vi "Test - 4.vi"() -> ()   [LabVIEW 2013]
uses:
  Channel/Ctls/ChannelSetting.ctl
  Channel/Ctls/IOType.ctl
  Channel/Ctls/Dimensions.ctl
  Section/Section.lvclass
  Channel/Channel.lvclass
  Generic/Generic.lvclass
  Item/Item.lvclass
  Item/Ctls/Item Reference.ctl
  <vilib>/NI Veristand/Custom Device API/Custom Device API.lvlib
panel:
  out "Property Names 2":string[](array[string])
  out "x = y?":bool
  out "PathName 2":string
  out "TagGUID":string
  out "Description":string
  out "PathName":string
  out "Property Names":string[](array[string])
  out "x-y":u32
  out "Request invalid?":bool
  out "Channels":T4(array[cluster])
  out "数组":T5(array[cluster])
  out "Value 2":variant
  # "19999"
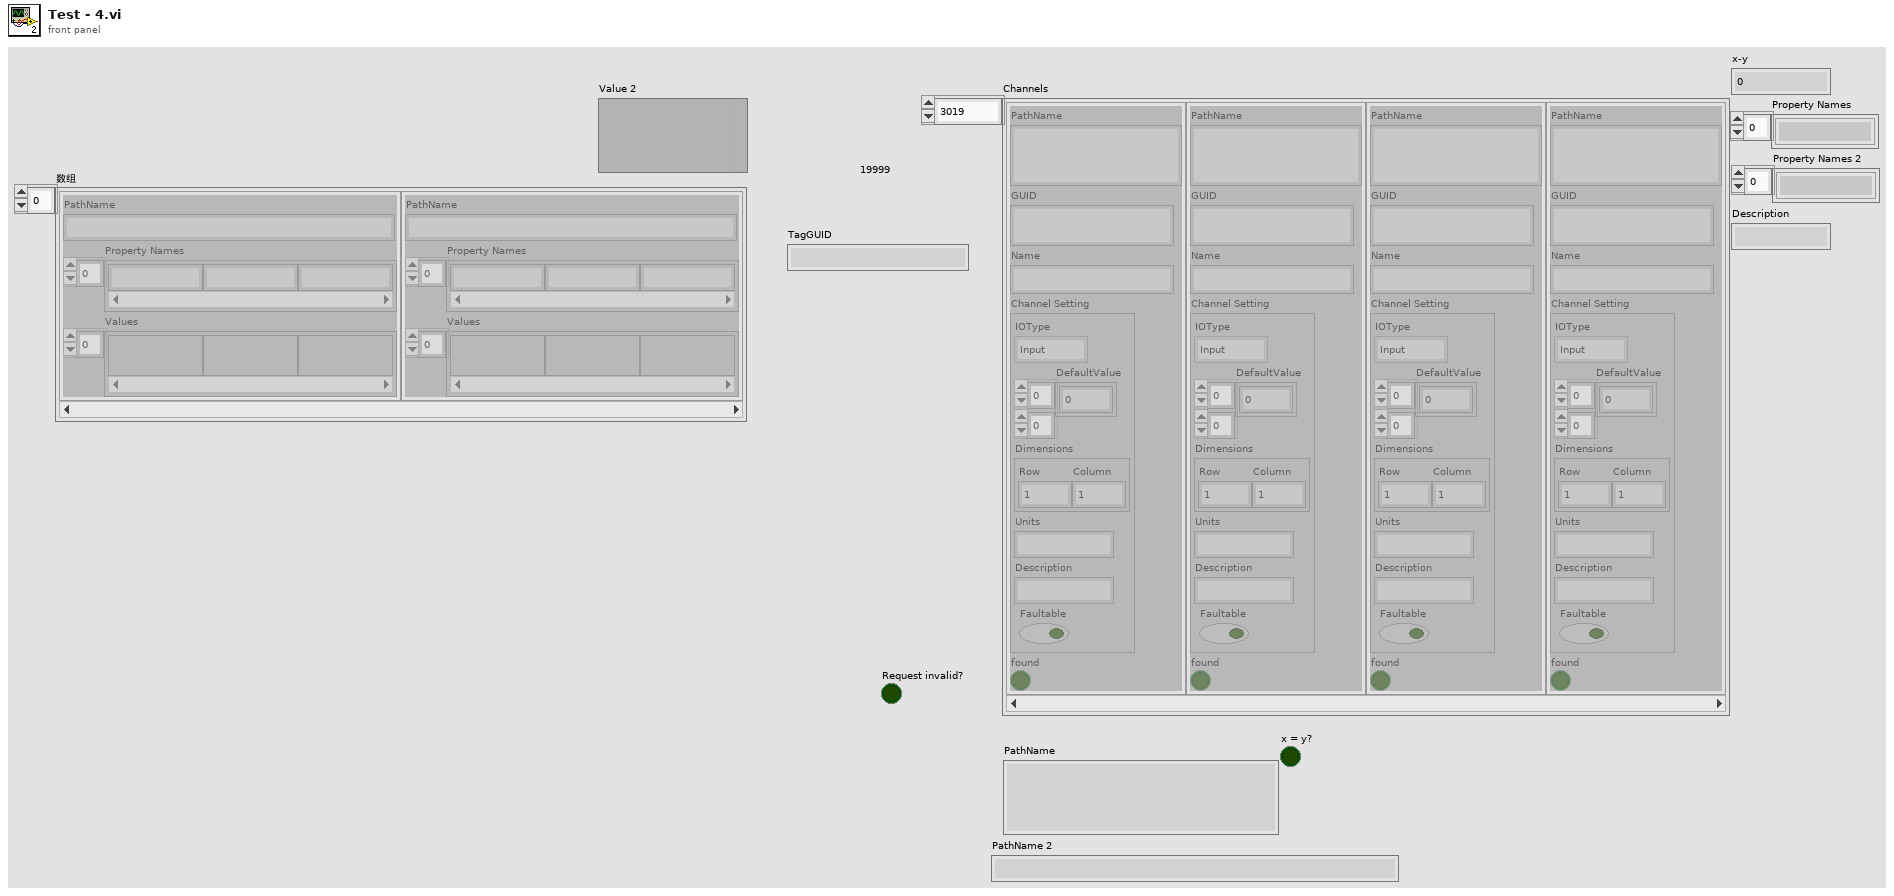
[diagram p1: front panel]
types:
  T1 = typedef "Hierarchy Framework.lvlib/Channel.lvclass/ChannelSetting.ctl" = cluster{"IOType":T2, "DefaultValue":dbl[][], "Dimensions":T3, "Units":string, "Description":string, "Faultable":bool}
  T2 = typedef "Hierarchy Framework.lvlib/Channel.lvclass/IOType.ctl" = enum16{"Input", "Output"}
  T3 = typedef "Hierarchy Framework.lvlib/Channel.lvclass/Dimensions.ctl" = cluster{"Row":i32, "Column":i32}
  T4 = cluster{"PathName":string, "GUID":string, "Name":string, "Channel Setting":T1, "found":bool}[]
  T5 = cluster{"PathName":string, "Property Names":string[], "Values":variant[]}[]
  T6 = typedef "Hierarchy Framework.lvlib/Item.lvclass/Item Reference.ctl" = u64
  T7 = cluster{"Accessors:PathName":string, "Property Names":string[], "Values":variant[]}
  T8 = cluster{"PathName":string, "GUID":string, "Name":string, "ChannelSetting":T1, "found":bool}
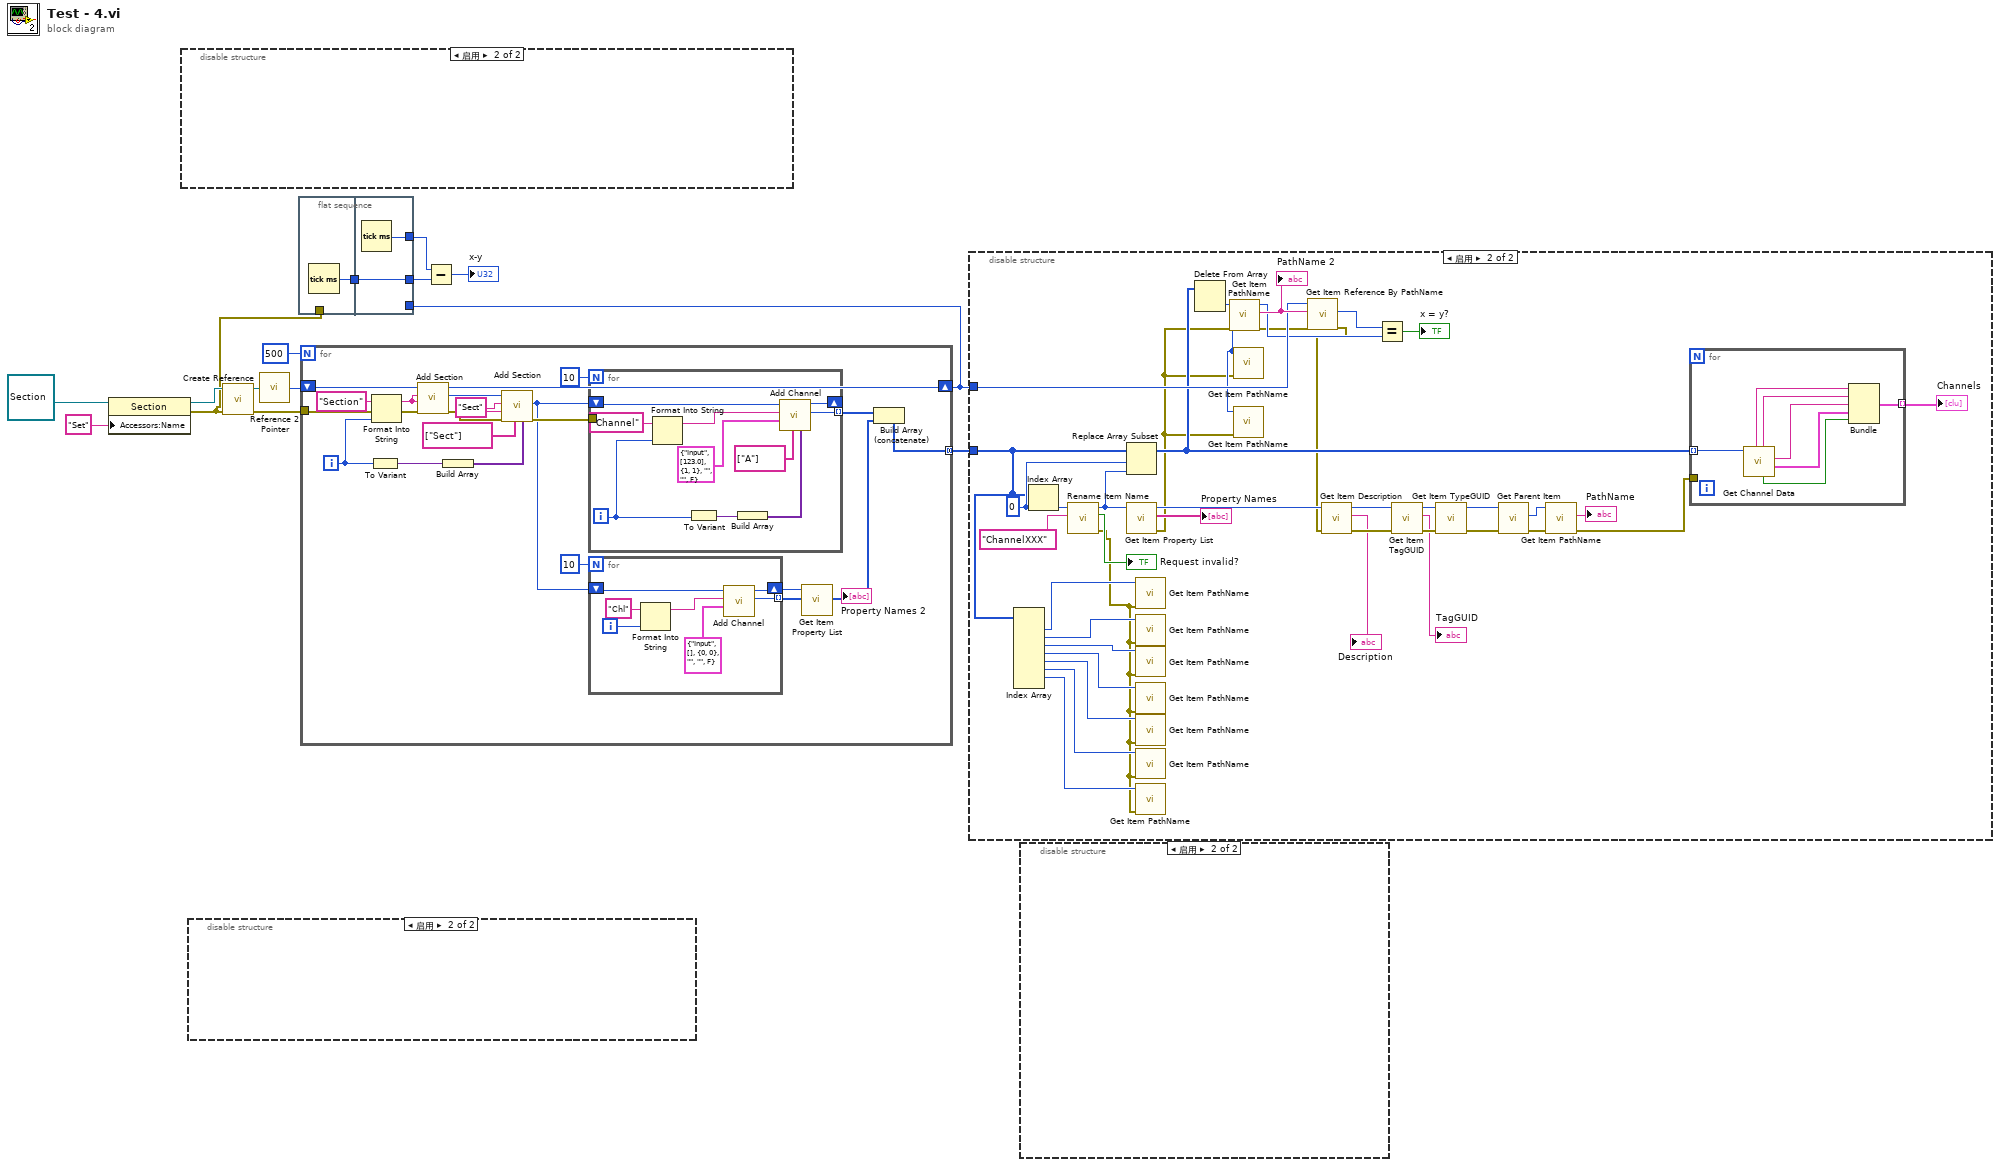
[diagram p0: block diagram]
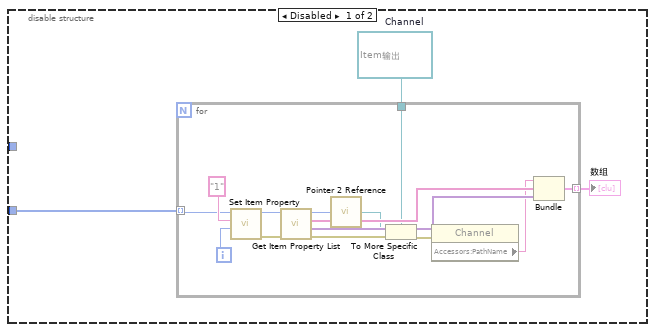
[diagram p2: hidden frame]
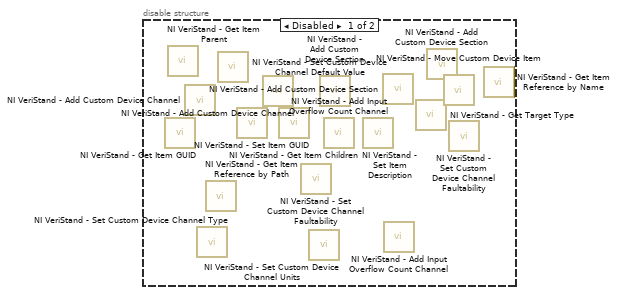
[diagram p3: hidden frame]
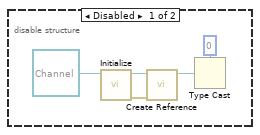
[diagram p4: hidden frame]
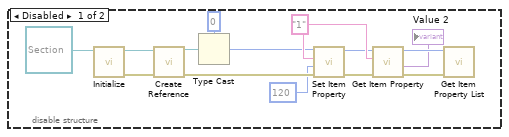
[diagram p5: hidden frame]
diagram:
  n1 = property class="Section"(reference=refnum<class "Section.lvclass"> refnum ("Framework.lvlib:Section"), "Accessors:Name"="Set" ("Name")) -> (reference out=w12:refnum<class "Section.lvclass">, error out=w8:errorcluster)  [unwired: 1 in]
  n2 = disable-structure shown="启用" {
    frame Disabled {
      n3 = call-dynamic "Initialize.vi"("Channel输入"=refnum<class "Channel.lvclass"> refnum ("Framework.lvlib:Channel")) -> ("error out"=w17:errorcluster, "Channel输出"=w18:refnum<class "Channel.lvclass">)  [unwired: 9 in]
      n4 = call "Create Reference.vi"("error in (no error)"=w17, "Generic"=w18) -> ("Generic Reference"=w16:refnum<data-value>)  [unwired: 8 in, 1 out]
      n5 = Type Cast(type=T6 0 ("Item Reference out"), x=w16) -> ()  [unwired: 1 out]
    }
    frame Enabled {
    }
  }
  n6 = disable-structure shown="启用" {
    frame Disabled {
      w31 = "1" ("Property Name")
      n7 = call-dynamic "Initialize.vi"("Section输入"=refnum<class "Section.lvclass"> refnum ("Framework.lvlib:Section")) -> ("error out"=w23:errorcluster, "Section输出"=w24:refnum<class "Section.lvclass">)  [unwired: 9 in]
      n8 = call "Create Reference.vi"("error in (no error)"=w23, "Generic"=w24) -> ("error out"=w29:errorcluster, "Generic Reference"=w21:refnum<data-value>)  [unwired: 8 in]
      n9 = Type Cast(type=T6 0 ("Item Reference out"), x=w21) -> (*(type *) &x=w20:T6)
      n10 = call "Set Item Property.vi"("error in (no error)"=w29, "Value"=u64 120 ("Generic Reference"), "Property Name"=w31, "Item Reference in"=w20) -> ("error out"=w28:errorcluster, "Item Reference out"=w30:T6)  [unwired: 5 in, 1 out]
      n11 = call "Get Item Property.vi"("error in (no error)"=w28, "Property Name"=w31, "Item Reference in"=w30) -> ("error out"=w27:errorcluster, "Value"=→"Value 2":variant, "Item Reference out"=w32:T6)  [unwired: 5 in, 1 out]
      n12 = call "Get Item Property List.vi"("error in (no error)"=w27, "Item Reference in"=w32) -> ()  [unwired: 6 in, 4 out]
    }
    frame Enabled {
    }
  }
  n13 = call "Create Reference.vi"("error in (no error)"=w8, "Generic"=w12) -> ("error out"=w14:errorcluster, "Generic Reference"=w10:refnum<data-value>)  [unwired: 8 in]
  n14 = call "Reference 2 Pointer.vi"("Generic Reference"=w10) -> ("Pointer"=w9:u64)  [unwired: 1 out]
  n15 = flat-sequence {
    tunnel: w8 -> [_]
    tunnel: [w34] -> w7
    tunnel: w3 -> [_]
    tunnel: w7 -> [w36]
    tunnel: [w36] -> w5
    tunnel: [w35] -> w6
    frame #0 {
      n16 = Tick Count (ms)() -> (millisecond timer value=w34:u32)
    }
    frame #1 {
      n17 = Tick Count (ms)() -> (millisecond timer value=w35:u32)
    }
  }
  n18 = for {
    N: 500 -> [_]
    tunnel: w14 -> [w49]
    shift-right: [w57] -> w3
    shift-left: w9 -> [w58]
    tunnel: [w51] -> w13 mode=concatenating
    i -> [w44]
    w38 = "Sect" ("SectionName")
    n19 = To Variant(anything=w44) -> (Variant=w43:variant)
    n20 = Format Into String(initial string="Section" ("初始字符串"), error in=w49, w44) -> (resulting string=w37:string, error out=w48:errorcluster)  [unwired: 1 in]
    n21 = call "Add Section.vi"("error in (no error)"=w48, "TypeGUID"=w37, "SectionName"=w37, "Section Reference in"=w58) -> ("error out"=w47:errorcluster, "Section Reference"=w53:u64, "Section Reference out"=w57:u64)  [unwired: 4 in, 1 out]
    n22 = Build Array(w43) -> (w42:variant[])
    n23 = call "Add Section.vi"("Property Values"=w42, "Property names"=string[] ["Sect"], "error in (no error)"=w47, "TypeGUID"=w38, "SectionName"=w38, "Section Reference in"=w53) -> ("error out"=w46:errorcluster, "Section Reference"=w41:u64)  [unwired: 2 in, 2 out]
    n24 = for {
      N: 10 -> [_]
      shift-right: [w74] -> _
      shift-left: w41 -> [w75]
      tunnel: [w71] -> w55 mode=indexing
      tunnel: w46 -> [_]
      i -> [w68]
      n25 = Format Into String(initial string="Channel" ("初始字符串"), w68) -> (resulting string=w73:string)  [unwired: 2 in, 1 out]
      n26 = To Variant(anything=w68) -> (Variant=w67:variant)
      n27 = Build Array(w67) -> (w66:variant[])
      n28 = call "Add Channel.vi"("Property Values"=w66, "Property names"=string[] ["A"], "Channel Setting"=T1 {"IOType"=enum."Input", "DefaultValue"=[[123.0]], "Dimensions"={"Row"=1, "Column"=1}, "Units"="", "Description"="", "Faultable"=FALSE} ("ChannelSetting"), "Channel Name"=w73, "Section Reference in"=w75) -> ("Channel Reference"=w71:u64, "Section Reference out"=w74:u64)  [unwired: 3 in, 2 out]
    }
    n29 = for {
      N: 10 -> [_]
      shift-right: [w64] -> w40
      shift-left: w41 -> [w65]
      tunnel: [w60] -> w50 mode=indexing
      i -> [w63]
      n30 = Format Into String(initial string="Chl" ("初始字符串"), w63) -> (resulting string=w62:string)  [unwired: 2 in, 1 out]
      n31 = call "Add Channel.vi"("Channel Setting"=T1 {"IOType"=enum."Input", "DefaultValue"=[], "Dimensions"={"Row"=0, "Column"=0}, "Units"="", "Description"="", "Faultable"=FALSE} ("ChannelSetting"), "Channel Name"=w62, "Section Reference in"=w65) -> ("Channel Reference"=w60:u64, "Section Reference out"=w64:u64)  [unwired: 5 in, 2 out]
    }
    n32 = call "Get Item Property List.vi"("Item Reference in"=w40) -> ("Property Names"=→"Property Names 2":string[])  [unwired: 7 in, 3 out]
    n33 = Build Array (concatenate)(w55, w50) -> (w51:u64[])
  }
  n34 = Subtract(x=w6, y=w5) -> (x-y=→"x-y":u32)
  n35 = disable-structure shown="启用" {
    disable-tunnel: w13 -> [w78 w103]
    disable-tunnel: w3 -> [_ w111]
    frame Disabled {
      w77 = refnum<data-value> refnum  # Channel
      n36 = for {
        tunnel: w78 -> [w90] mode=indexing
        tunnel: w77 -> [w82]
        tunnel: [w79] -> w76 mode=indexing
        i -> [w89]
        n37 = call "Set Item Property.vi"("Value"=w89, "Property Name"="1", "Item Reference in"=w90) -> ("error out"=w92:errorcluster, "Item Reference out"=w93:T6)  [unwired: 6 in, 1 out]
        n38 = call "Get Item Property List.vi"("error in (no error)"=w92, "Item Reference in"=w93) -> ("error out"=w81:errorcluster, "Values"=w87:variant[], "Property Names"=w88:string[], "Item Reference out"=w83:T6)  [unwired: 6 in]
        n39 = call "Pointer 2 Reference.vi"("Pointer"=w83) -> ("Generic Reference"=w84:refnum<data-value>)  [unwired: 1 out]
        n40 = To More Specific Class(target class=w82, reference=w84, error in=w81) -> (specific class reference=w86:refnum<data-value>, error out=w85:errorcluster)
        n41 = property class="Channel"(reference=w86, error in=w85) -> ("Accessors:PathName"=w80:string)  [unwired: 2 out]
        n42 = Bundle("Accessors:PathName"=w80, "Property Names"=w88, "Values"=w87) -> (w79:T7)  [unwired: 1 in]
      }
      "数组" <- w76
    }
    frame Enabled {
      w128 = 0 ("索引")
      n43 = Index Array(array=w103) -> (element #1=w102:u64, element #2=w101:u64, element #3=w100:u64, element #4=w99:u64, element #5=w98:u64, element #6=w97:u64, element #7=w96:u64)  [unwired: 8 in, 1 out]
      n44 = Index Array(array=w103, index=w128) -> (element=w129:u64)
      n45 = call "Rename Item Name.vi"("New Name"="ChannelXXX", "Item Reference in"=w129) -> ("error out"=w95:errorcluster, "Request invalid?"=→"Request invalid?":bool, "Item Reference out"=w127:T6)  [unwired: 7 in]
      n46 = Replace Array Subset(array=w103, new element=w127, index=w128) -> (w107:u64[])
      n47 = call "Get Item Property List.vi"("Item Reference in"=w127) -> ("error out"=w94:errorcluster, "Property Names"=→"Property Names":string[], "Item Reference out"=w125:T6)  [unwired: 7 in, 1 out]
      n48 = call "Get Item PathName.vi"("error in (no error)"=w95, "Item Reference in"=w102) -> ()  [unwired: 6 in, 4 out]
      n49 = call "Get Item PathName.vi"("error in (no error)"=w95, "Item Reference in"=w101) -> ()  [unwired: 6 in, 4 out]
      n50 = call "Get Item PathName.vi"("error in (no error)"=w95, "Item Reference in"=w100) -> ()  [unwired: 6 in, 4 out]
      n51 = call "Get Item PathName.vi"("error in (no error)"=w95, "Item Reference in"=w99) -> ()  [unwired: 6 in, 4 out]
      n52 = call "Get Item PathName.vi"("error in (no error)"=w95, "Item Reference in"=w98) -> ()  [unwired: 6 in, 4 out]
      n53 = call "Get Item PathName.vi"("error in (no error)"=w95, "Item Reference in"=w97) -> ()  [unwired: 6 in, 4 out]
      n54 = call "Get Item PathName.vi"("error in (no error)"=w95, "Item Reference in"=w96) -> ()  [unwired: 6 in, 4 out]
      n55 = Delete From Array(array=w107) -> (deleted portion=w104:u64)  [unwired: 2 in, 1 out]
      n56 = call "Get Item PathName.vi"("error in (no error)"=w94, "Item Reference in"=w104) -> ("error out"=w106:errorcluster, "PathName"=w112:string, "Item Reference out"=w109:T6)  [unwired: 6 in, 1 out]
      "PathName 2" <- w112
      n57 = call "Get Item PathName.vi"("error in (no error)"=w94, "Item Reference in"=w104) -> ()  [unwired: 6 in, 4 out]
      n58 = call "Get Item PathName.vi"("error in (no error)"=w94, "Item Reference in"=w104) -> ()  [unwired: 6 in, 4 out]
      n59 = call "Get Item Reference By PathName.vi"("error in (no error)"=w106, "Item PathName"=w112, "Root Item Reference in"=w111) -> ("error out"=w105:errorcluster, "Item Reference"=w110:u64)  [unwired: 5 in, 2 out]
      n60 = call "Get Item Description.vi"("error in (no error)"=w105, "Item Reference in"=w125) -> ("error out"=w121:errorcluster, "Description"=→"Description":string, "Item Reference out"=w124:T6)  [unwired: 6 in, 1 out]
      n61 = Equal?(x=w110, y=w109) -> (x = y?=→"x = y?":bool)
      n62 = call "Get Item TagGUID.vi"("error in (no error)"=w121, "Item Reference in"=w124) -> ("error out"=w122:errorcluster, "TagGUID"=→"TagGUID":string, "Item Reference out"=w123:T6)  [unwired: 6 in, 1 out]
      n63 = call "Get Item TypeGUID.vi"("error in (no error)"=w122, "Item Reference in"=w123) -> ("error out"=w119:errorcluster, "Item Reference out"=w120:T6)  [unwired: 6 in, 2 out]
      n64 = call "Get Parent Item.vi"("error in (no error)"=w119, "Item Reference in"=w120) -> ("error out"=w116:errorcluster, "Parent Item Reference"=w118:u64)  [unwired: 6 in, 2 out]
      n65 = call "Get Item PathName.vi"("error in (no error)"=w116, "Item Reference in"=w118) -> ("error out"=w113:errorcluster, "PathName"=→"PathName":string)  [unwired: 6 in, 2 out]
      n66 = for {
        tunnel: w107 -> [w139] mode=indexing
        tunnel: [w134] -> w132 mode=indexing
        tunnel: w113 -> [_]
        n67 = call "Get Channel Data.vi"("Channel Reference in"=w139) -> ("ChannelSetting"=w135:T1, "Name"=w136:string, "found"=w133:bool, "GUID"=w137:string, "PathName"=w138:string)  [unwired: 4 in, 2 out]
        n68 = Bundle("PathName"=w138, "GUID"=w137, "Name"=w136, "ChannelSetting"=w135, "found"=w133) -> (w134:T8)  [unwired: 1 in]
      }
      "Channels" <- w132
    }
  }
  n69 = disable-structure shown="启用" {
    frame Disabled {
      n70 = call <vilib>:"NI VeriStand - Get Item GUID.vi"() -> ()  [unwired: 9 in, 3 out]
      n71 = call <vilib>:"NI VeriStand - Get Item Parent.vi"() -> ()  [unwired: 8 in, 4 out]
      n72 = call <vilib>:"NI VeriStand - Add Custom Device Channel.vi"() -> ()  [unwired: 8 in, 4 out]
      n73 = call <vilib>:"NI VeriStand - Set Custom Device Channel Type.vi"() -> ()  [unwired: 10 in, 2 out]
      n74 = call <vilib>:"NI VeriStand - Get Item Reference by Path.vi"() -> ()  [unwired: 8 in, 4 out]
      n75 = call <vilib>:"NI VeriStand - Set Custom Device Channel Default Value.vi"() -> ()  [unwired: 10 in, 2 out]
      n76 = call <vilib>:"NI VeriStand - Set Item GUID.vi"() -> ()  [unwired: 10 in, 2 out]
      n77 = call <vilib>:"NI VeriStand - Add Custom Device Channel.vi"() -> ()  [unwired: 8 in, 4 out]
      n78 = call <vilib>:"NI VeriStand - Get Item Children.vi"() -> ()  [unwired: 8 in, 4 out]
      n79 = call <vilib>:"NI VeriStand - Set Custom Device Channel Faultability.vi"() -> ()  [unwired: 10 in, 2 out]
      n80 = call <vilib>:"NI VeriStand - Set Custom Device Channel Units.vi"() -> ()  [unwired: 10 in, 2 out]
      n81 = call <vilib>:"NI VeriStand - Add Custom Device Section.vi"() -> ()  [unwired: 8 in, 4 out]
      n82 = call <vilib>:"NI VeriStand - Add Input Overflow Count Channel.vi"() -> ()  [unwired: 9 in, 3 out]
      n83 = call <vilib>:"NI VeriStand - Set Item Description.vi"() -> ()  [unwired: 9 in, 3 out]
      n84 = call <vilib>:"NI VeriStand - Add Custom Device Section.vi"() -> ()  [unwired: 8 in, 4 out]
      n85 = call <vilib>:"NI VeriStand - Add Input Overflow Count Channel.vi"() -> ()  [unwired: 9 in, 3 out]
      n86 = call <vilib>:"NI VeriStand - Get Target Type.vi"() -> ()  [unwired: 9 in, 3 out]
      n87 = call <vilib>:"NI VeriStand - Add Custom Device Section.vi"() -> ()  [unwired: 8 in, 4 out]
      n88 = call <vilib>:"NI VeriStand - Move Custom Device Item.vi"() -> ()  [unwired: 9 in, 3 out]
      n89 = call <vilib>:"NI VeriStand - Set Custom Device Channel Faultability.vi"() -> ()  [unwired: 10 in, 2 out]
      n90 = call <vilib>:"NI VeriStand - Get Item Reference by Name.vi"() -> ()  [unwired: 8 in, 4 out]
    }
    frame Enabled {
    }
  }
